vi "main.vi"(8 "Error in":errorcluster) -> (0 "Error out":errorcluster)   [LabVIEW 2018, in "Controller.lvlib"]
uses:
  Controller.lvlib
  Common/Common.lvlib
  ctl/Module Queue - Action.ctl
  ctl/Module - State.ctl
  Common/ctl/Stop All - Action.ctl
  Error Handler/Error Handler.lvlib
  Error Handler/ctl/Module - State.ctl
  Sensor Interface/Sensor Interface.lvlib
  Display Console/Display Console.lvlib
  User Console/User Console.lvlib
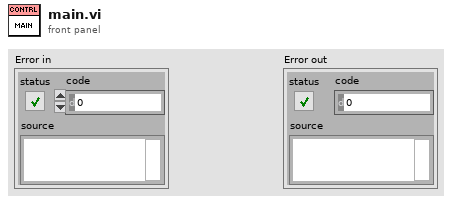
[diagram p1: front panel]
types:
  T1 = typedef "Controller.lvlib/Module Queue - Action.ctl" = enum16{"Create", "Get", "Destroy"}
  T2 = typedef "Common.lvlib/Stop All - Action.ctl" = enum16{"Create", "Fire", "Get", "Destroy"}
  T3 = typedef "Controller.lvlib/Module - State.ctl" = enum16{"Init", "Idle", "Error", "Close"}
  T4 = typedef "Error Handler.lvlib/Module - State.ctl" = enum16{"Init", "Idle", "Error", "Close", "Handle External Error", "Log Error"}
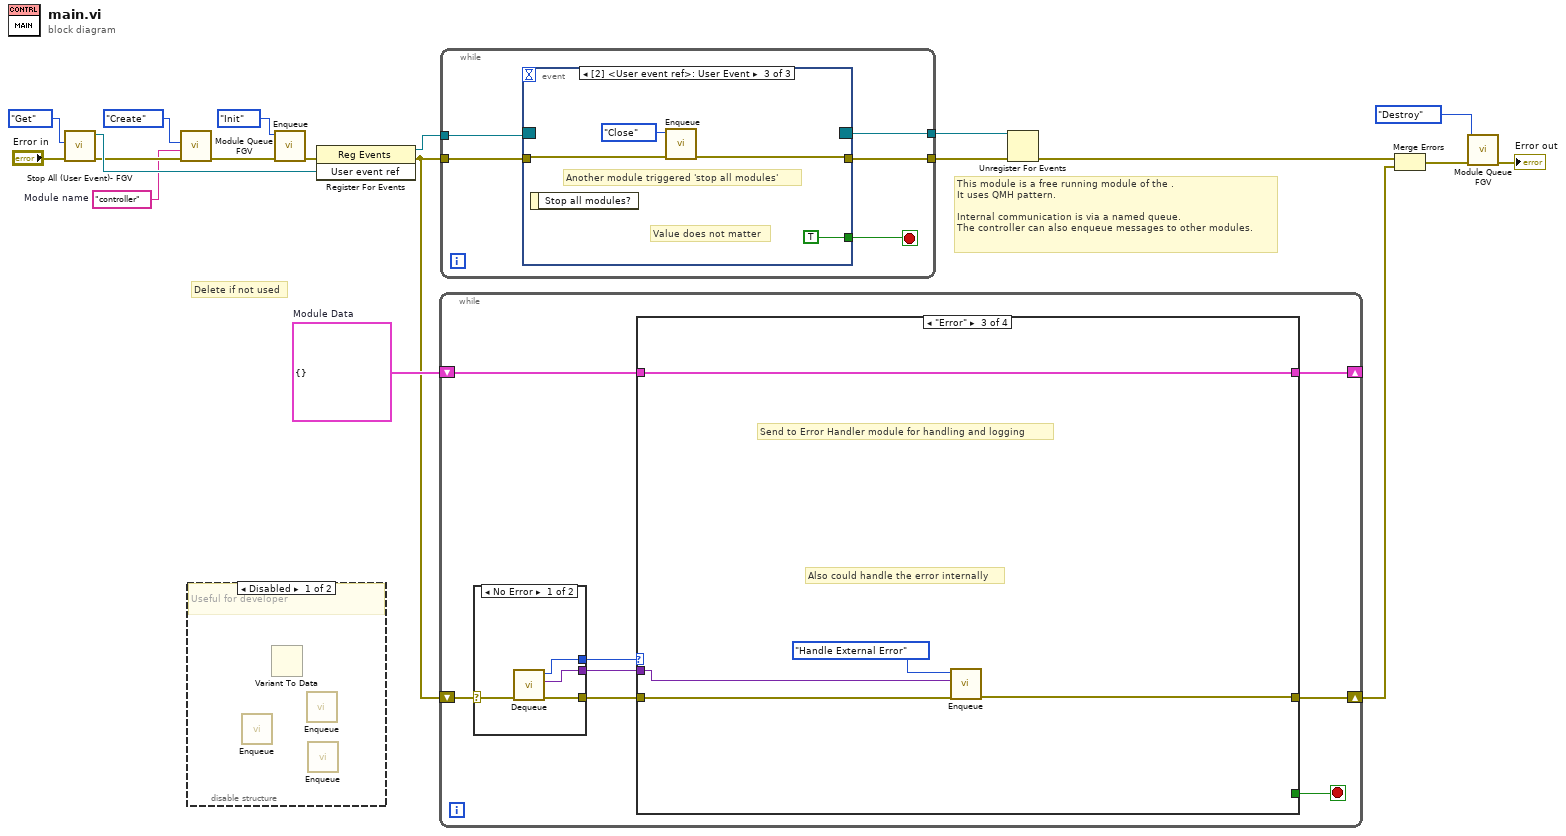
[diagram p0: block diagram]
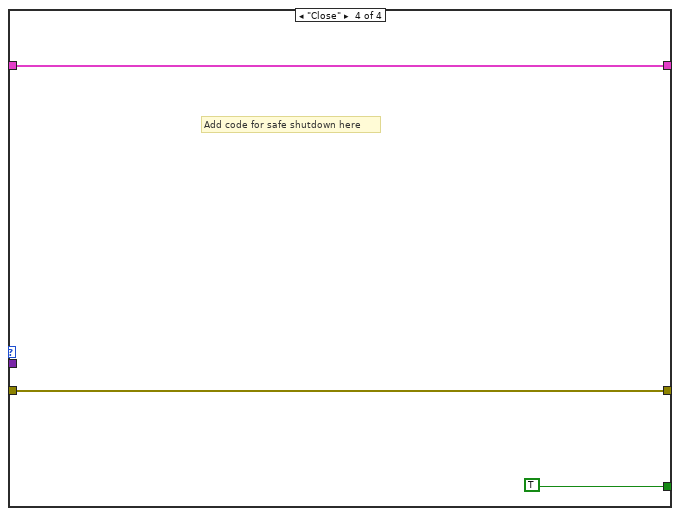
[diagram p4: hidden frame]
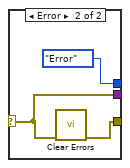
[diagram p5: hidden frame]
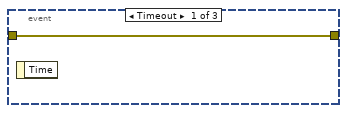
[diagram p7: hidden frame]
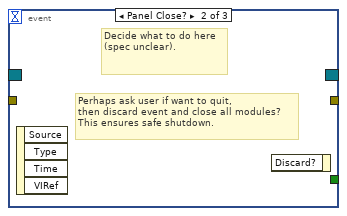
[diagram p8: hidden frame]
diagram:
  w1 = "controller"  # Module name
  w8 = cluster{} {}  # Module Data
  # "This module is a free running module of the .\nIt uses QMH pattern.\n\nInternal communication is via a named queue.\nThe controller can also enqueue messages to other modules."
  # "Delete if not used"
  n1 = call "Stop All (User Event)- FGV.vi"("error in"="Error in", "Action"=Stop_All_-_Action."Get") -> ("error out"=w10:errorcluster, "User event ref"=w15:refnum<user-event>)  [unwired: 8 in]
  n2 = call "Module Queue FGV.vi"("Error in"=w10, "Queue name"=w1, "Action"=Module_Queue_-_Action."Create") -> ("Error out"=w18:errorcluster)  [unwired: 7 in, 1 out]
  n3 = disable-structure shown="Disabled" {
    frame Disabled {
      # "Useful for developer"
      n4 = call "Enqueue.vi"() -> ()  [unwired: 11 in, 1 out]
      n5 = Variant To Data() -> ()  [unwired: 3 in, 2 out]
      n6 = call "Enqueue.vi"() -> ()  [unwired: 11 in, 1 out]
      n7 = call "Enqueue.vi"() -> ()  [unwired: 11 in, 1 out]
    }
    frame Enabled {
    }
  }
  n8 = call "Enqueue.vi"("error in (no error)"=w18, "State"=Module_-_State."Init") -> ("error out"=w9:errorcluster)  [unwired: 9 in]
  n9 = register-events(error in=w9, w15) -> (reference out=w13:refnum<event-registration>, error out=w3:errorcluster)  [unwired: 1 in]
  n10 = while {
    shift-right: [w27] -> _
    shift-left: w8 -> [w26]
    shift-right: [w20] -> w2
    shift-left: w3 -> [w25]
    stop <- w21 stop-if-true
    n11 = case shown="No Error" w25 {
      selector: w25 -> [w42 w44]
      tunnel: [w41 Module_-_State."Error" ("State")] -> w24
      tunnel: [w40 w44] -> w23
      tunnel: [w39 w43] -> w22
      frame No Error {
        n12 = call "Dequeue.vi"("error in"=w42) -> ("error out"=w39:errorcluster, "Data"=w40:variant, "State"=w41:T3)  [unwired: 8 in]
      }
      frame Error {
        # "Instead of dequeue,\nhandle the error"
        n13 = call <vilib>:"Clear Errors.vi"("error in (no error)"=w44) -> ("error out"=w43:errorcluster)  [unwired: 5 in, 1 out]
      }
    }
    n14 = case shown="\"Error\"" w24 {
      tunnel: [w28 w30 w35 w36] -> w27
      tunnel: w26 -> [w28 w30 w35 w36]
      tunnel: w23 -> [_ _ w32 _]
      tunnel: w22 -> [_ w29 w34 w37]
      tunnel: [_ _ _ TRUE] -> w21
      tunnel: [_ w29 w33 w37] -> w20
      frame "Init", Default {
      }
      frame "Idle" {
      }
      frame "Error" {
        # "Send to Error Handler module for handling and logging"
        # "Also could handle the error internally"
        n15 = call "Enqueue.vi"("error in (no error)"=w34, "Data"=w32, "State"=Module_-_State."Handle External Error") -> ("error out"=w33:errorcluster)  [unwired: 8 in]
      }
      frame "Close" {
        # "Add code for safe shutdown here"
      }
    }
  }
  n16 = while {
    tunnel: w13 -> [w50]
    tunnel: [w49] -> w12
    tunnel: w3 -> [w48]
    tunnel: [w47] -> w11
    stop <- w46 stop-if-true
    n17 = event shown="[2] <User event ref>: User Event" {
      selector: w50 -> [_ _ _]
      dyn-events: [_ _ _] -> w49
      timeout: _ -> [_ _ _]
      tunnel: w48 -> [w51 _ w55]
      tunnel: [w51 _ w54] -> w47
      tunnel: [_ _ TRUE] -> w46
      event Timeout {
        n18 = event-data() -> ()  [unwired: 1 in, 1 out]
      }
      event Panel Close? {
        # "Perhaps ask user if want to quit,\nthen discard event and close all modules?\nThis ensures safe shutdown."
        # "Decide what to do here\n(spec unclear)."
        n19 = event-data() -> ()  [unwired: 1 in, 4 out]
        n20 = event-data() -> ()  [unwired: 2 in, 1 out]
      }
      event User Event {
        # "Value does not matter"
        # "Another module triggered 'stop all modules'"
        n21 = event-data() -> ()  [unwired: 1 in, 1 out]
        n22 = call "Enqueue.vi"("error in (no error)"=w55, "State"=Module_-_State."Close") -> ("error out"=w54:errorcluster)  [unwired: 9 in]
      }
    }
  }
  n23 = Unregister For Events(event registration refnum=w12, error in=w11) -> (error out=w7:errorcluster)
  n24 = Merge Errors(w7, w2) -> (w6:errorcluster)
  n25 = call "Module Queue FGV.vi"("Error in"=w6, "Action"=Module_Queue_-_Action."Destroy") -> ("Error out"=→"Error out":errorcluster)  [unwired: 8 in, 1 out]
